vi "Filter ECAT Path by Object Index.vi"(10 "Object Index In":i32, 11 "ECAT Variable Path In":string) -> (2 "Found":bool, 3 "Variable Name":string)   [LabVIEW 2016]
panel:
  in  "regular expression":string="[~0-9~\\\\\\\\]+_%d_[0-9]"
  # "NI-ECAT\\EtherCAT Master\\Device4\\^NoModule^\\Inputs_6656\\Status word_24641_0"
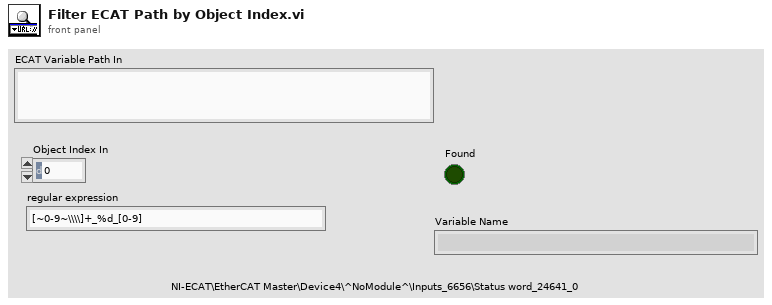
[diagram p1: front panel]
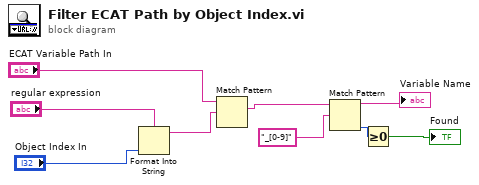
[diagram p0: block diagram]
diagram:
  n1 = Format Into String(format string="regular expression", "Object Index In") -> (resulting string=w1:string)  [unwired: 2 in, 1 out]
  n2 = Match Pattern(string="ECAT Variable Path In", regular expression=w1) -> (match substring=w8:string)  [unwired: 1 in, 3 out]
  n3 = Match Pattern(string=w8, regular expression="_[0-9]") -> (before substring=→"Variable Name":string, offset past match=w3:i32)  [unwired: 1 in, 2 out]
  n4 = Greater Or Equal To 0?(x=w3) -> (x >= 0?=→"Found":bool)
